vi "Day08-02_모터 속도 변경.vi"() -> ()   [LabVIEW 2021]
uses:
  <vilib>/DAQmx/read.llb/DAQmx Read (Counter DBL 1Chan 1Samp).vi
  <vilib>/DAQmx/write.llb/DAQmx Write (Digital Bool 1Line 1Point).vi
  <vilib>/DAQmx/write.llb/DAQmx Write (Counter Frequency 1Chan 1Samp).vi
  <vilib>/DAQmx/create/channels.llb/DAQmx Create Channel (CO-Pulse Generation-Frequency).vi
  <vilib>/DAQmx/configure/timing.llb/DAQmx Timing (Implicit).vi
  <vilib>/DAQmx/create/channels.llb/DAQmx Create Channel (DO-Digital Output).vi
  <vilib>/DAQmx/create/channels.llb/DAQmx Create Channel (CI-Count Edges).vi
  <vilib>/DAQmx/miscellaneous.llb/DAQmx Fill In Error Info.vi
  <resource>/objmgr/daqmx.rc
panel:
  out "RPM":dbl
  in  "정회전":bool caption="데이터"
  in  "주기 점유율 2":dbl=0.1 min=0.1 max=0.9 step=0.1
  in  "정지 3":bool
  in  "정지 2":bool
  in  "주기 점유율":dbl=0.1 min=0.1 max=0.9 step=0.1
  in  "초기 지연":dbl format="%.6f"
  in  "정지":bool
  in  "주파수":dbl=1.0 format="%.6f"
  in  "주기 점유율":dbl=0.5 format="%.6f"
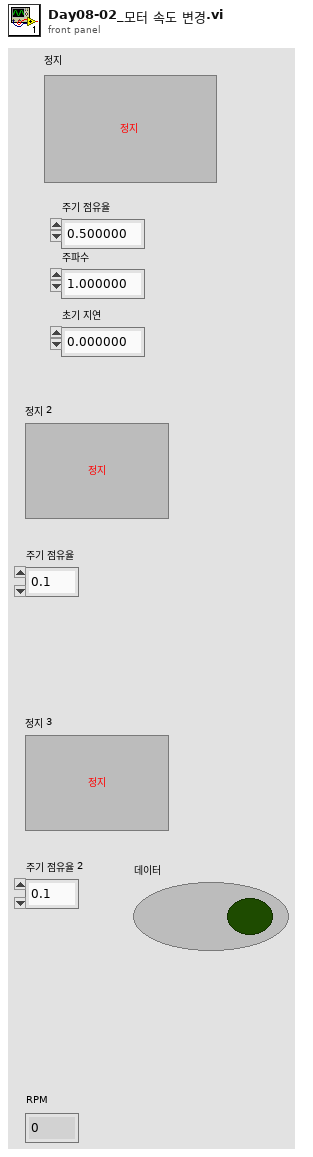
[diagram p1: front panel]
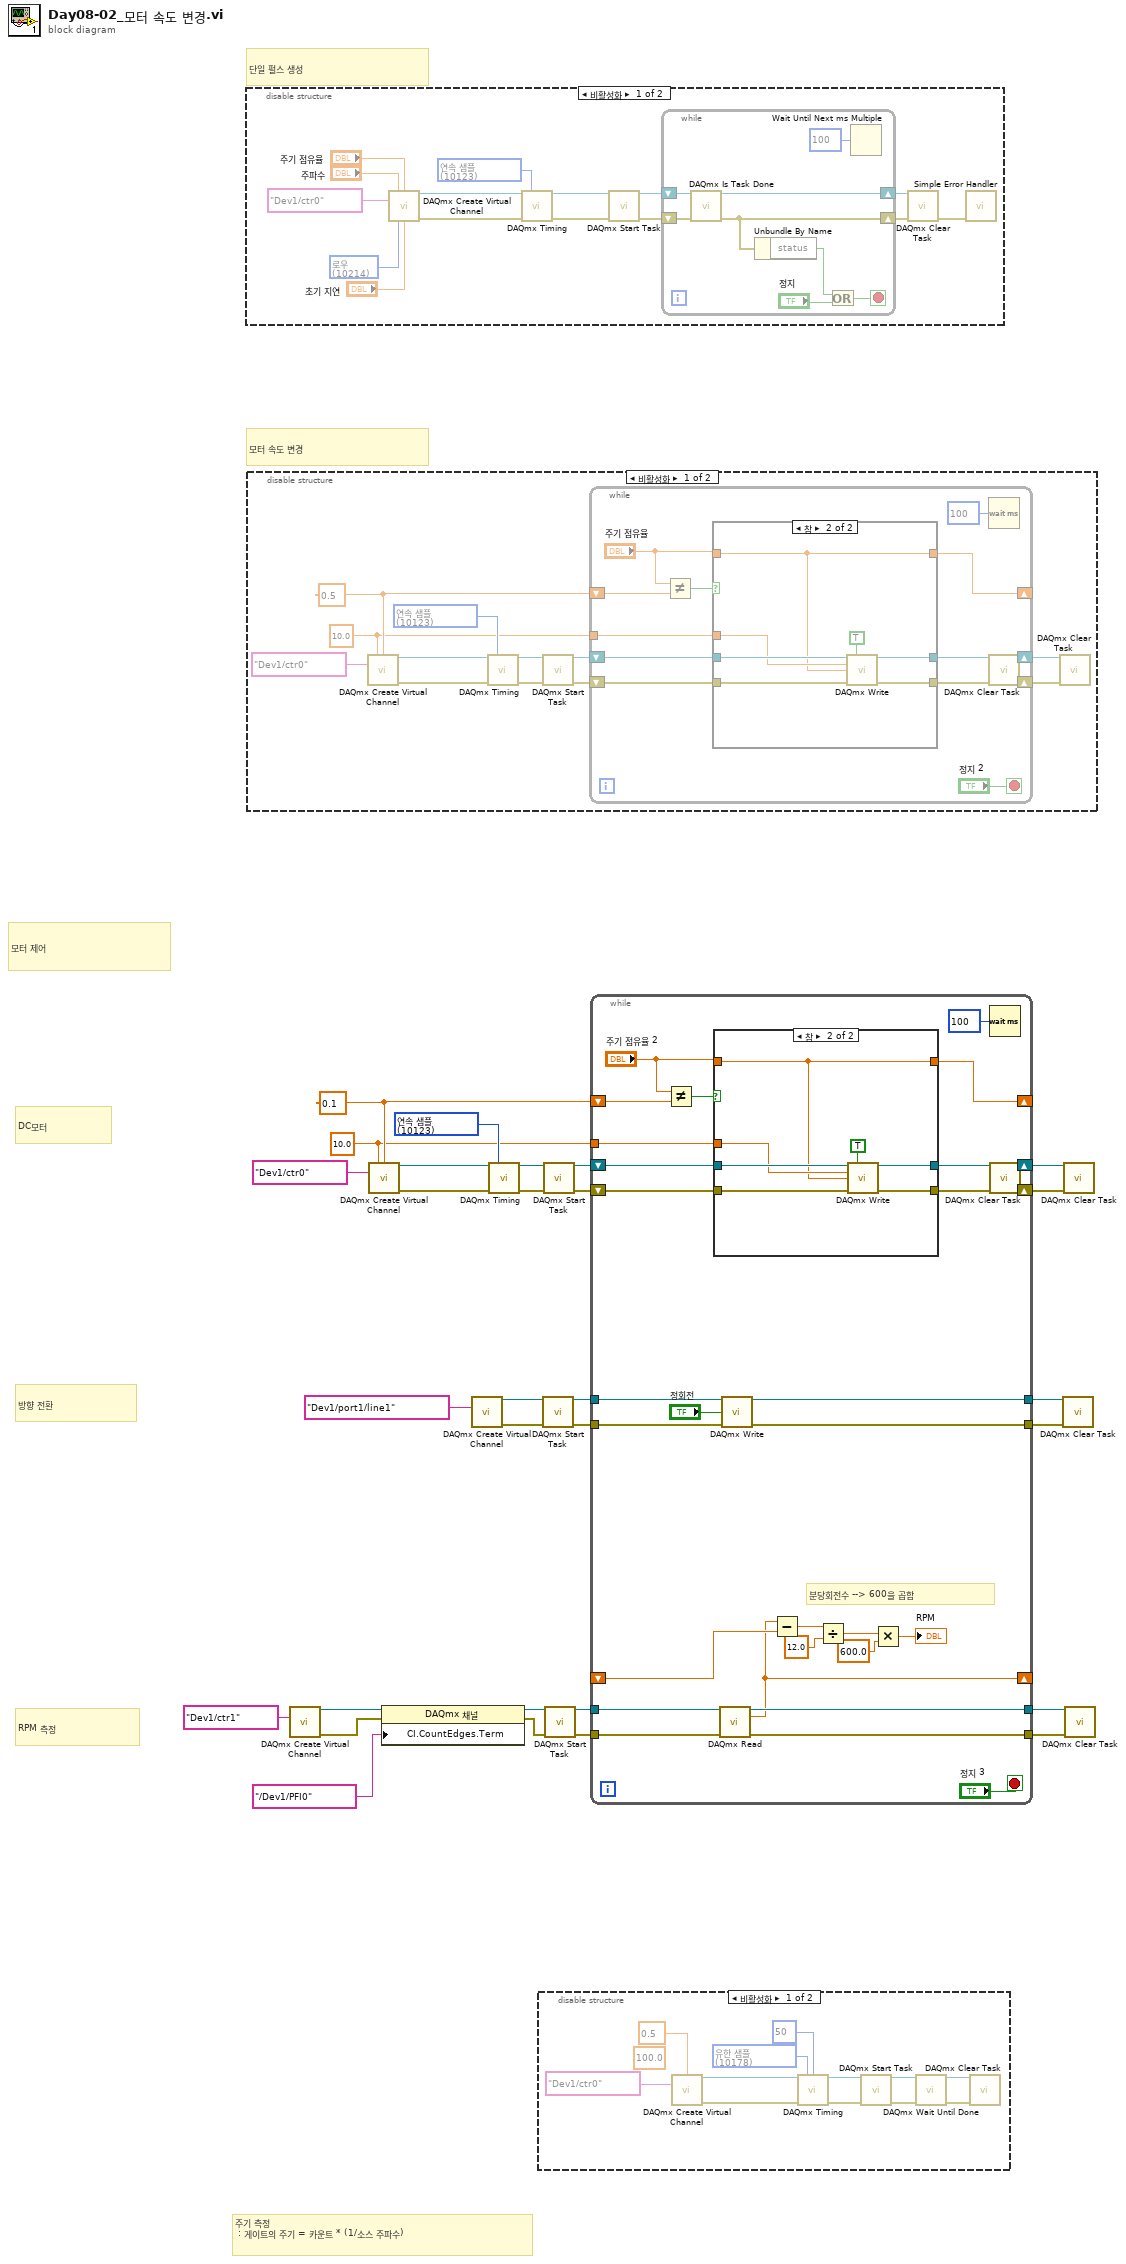
[diagram p0: block diagram]
diagram:
  w18 = 10.0
  w19 = 0.1
  w22 = 10123 items=["유한 샘플"=10178, "연속 샘플"=10123, "하드웨어 타이밍에 의한 단일 포인트"=12522] ("sample mode")
  # "RPM 측정"
  # "방향 전환"
  # "DC모터"
  # "주기 측정\n : 게이트의 주기 = 카운트 * (1/소스 주파수)"
  # "모터 제어"
  # "단일 펄스 생성"
  # "모터 속도 변경"
  n1 = disable-structure shown="비활성화" {
    frame Disabled {
      w34 = 10123 items=["유한 샘플"=10178, "연속 샘플"=10123, "하드웨어 타이밍에 의한 단일 포인트"=12522] ("sample mode")
      w36 = 10214 items=["하이"=10192, "로우"=10214] ("idle state")
      n2 = call-poly <vilib>:"DAQmx Create Virtual Channel.vi"("frequency"="주파수", "duty cycle"="주기 점유율", "counter"=tag "Dev1/ctr0", "idle state"=w36, "initial delay"="초기 지연") -> ("task out"=w44:refnum<k21>, "error out"=w43:errorcluster)  [unwired: 9 in]
      n3 = call-poly <vilib>:"DAQmx Timing.vi"("task/channels in"=w44, "sample mode"=w34, "error in"=w43) -> ("task out"=w42:refnum<k21>, "error out"=w41:errorcluster)  [unwired: 11 in]
      n4 = call <vilib>:"DAQmx Start Task.vi"("task/channels in"=w42, "error in"=w41) -> ("task out"=w40:refnum<k21>, "error out"=w39:errorcluster)  [unwired: 12 in]
      n5 = while {
        shift-right: [w50] -> w38
        shift-left: w40 -> [w52]
        shift-right: [w47] -> w37
        shift-left: w39 -> [w51]
        stop <- w48 stop-if-true
        n6 = call <vilib>:"DAQmx Is Task Done.vi"("task/channels in"=w52, "error in"=w51) -> ("task out"=w50:refnum<k21>, "error out"=w47:errorcluster)  [unwired: 11 in, 1 out]
        n7 = Unbundle By Name(w47) -> ("status"=w46:bool)
        n8 = Or(x=w46, y="정지") -> (x .or. y?=w48:bool)
        n9 = Wait Until Next ms Multiple(millisecond multiple=u32 100 ("ms 배수")) -> ()  [unwired: 1 out]
      }
      n10 = call <vilib>:"DAQmx Clear Task.vi"("task in"=w38, "error in"=w37) -> ("error out"=w33:errorcluster)  [unwired: 13 in]
      n11 = call <vilib>:"Simple Error Handler.vi"("error in (no error)"=w33) -> ()  [unwired: 4 in, 5 out]
    }
    frame Enabled {
    }
  }
  n12 = disable-structure shown="비활성화" {
    frame Disabled {
      w53 = 10.0
      w54 = 0.5
      w57 = 10123 items=["유한 샘플"=10178, "연속 샘플"=10123, "하드웨어 타이밍에 의한 단일 포인트"=12522] ("sample mode")
      n13 = call-poly <vilib>:"DAQmx Create Virtual Channel.vi"("frequency"=w53, "duty cycle"=w54, "counter"=tag "Dev1/ctr0") -> ("task out"=w64:refnum<k21>, "error out"=w63:errorcluster)  [unwired: 11 in]
      n14 = call-poly <vilib>:"DAQmx Timing.vi"("task/channels in"=w64, "sample mode"=w57, "error in"=w63) -> ("task out"=w62:refnum<k21>, "error out"=w61:errorcluster)  [unwired: 11 in]
      n15 = call <vilib>:"DAQmx Start Task.vi"("task/channels in"=w62, "error in"=w61) -> ("task out"=w60:refnum<k21>, "error out"=w59:errorcluster)  [unwired: 12 in]
      n16 = while {
        shift-right: [w73] -> w56
        shift-left: w60 -> [w75]
        shift-right: [w72] -> w55
        shift-left: w59 -> [w74]
        shift-right: [w65] -> _
        shift-left: w54 -> [w68]
        tunnel: w53 -> [w70]
        stop <- "정지 2" stop-if-true
        n17 = Not Equal?(x="주기 점유율", y=w68) -> (x != y?=w69:bool)
        n18 = case shown="참" w69 {
          tunnel: w75 -> [w77 w85]
          tunnel: w74 -> [w76 w84]
          tunnel: [w77 w83] -> w73
          tunnel: [w76 w82] -> w72
          tunnel: w70 -> [_ w80]
          tunnel: "주기 점유율" -> [w78 w79]
          tunnel: [w78 w79] -> w65
          frame False {
          }
          frame True {
            n19 = call-poly <vilib>:"DAQmx Write.vi"("task/channels in"=w85, "auto start"=TRUE, "frequency"=w80, "duty cycle"=w79, "error in"=w84) -> ("task out"=w83:refnum<k21>, "error out"=w82:errorcluster)  [unwired: 8 in, 1 out]
          }
        }
        n20 = Wait (ms)(milliseconds to wait=u32 100 ("대기 시간 (ms)")) -> ()  [unwired: 1 out]
      }
      n21 = call <vilib>:"DAQmx Clear Task.vi"("task in"=w56, "error in"=w55) -> ()  [unwired: 13 in, 1 out]
      n22 = call <vilib>:"DAQmx Clear Task.vi"("task in"=w56, "error in"=w55) -> ()  [unwired: 13 in, 1 out]
    }
    frame Enabled {
    }
  }
  n23 = call-poly <vilib>:"DAQmx Create Virtual Channel.vi"("counter"=tag "Dev1/ctr1") -> ("task out"=w10:refnum<k21>, "error out"=w3:errorcluster)  [unwired: 13 in]
  n24 = call-poly <vilib>:"DAQmx Create Virtual Channel.vi"("frequency"=w18, "duty cycle"=w19, "counter"=tag "Dev1/ctr0") -> ("task out"=w29:refnum<k21>, "error out"=w28:errorcluster)  [unwired: 11 in]
  n25 = property class="DAQmx 채널"(reference=w10, error in=w3, "CI.CountEdges.Term"=tag "/Dev1/PFI0" ("카운터 입력:에지 카운트:입력:터미널")) -> (reference out=w5:refnum<k21>, error out=w2:errorcluster)
  n26 = call-poly <vilib>:"DAQmx Create Virtual Channel.vi"("lines"=tag "Dev1/port1/line1") -> ("task out"=w17:refnum<k21>, "error out"=w16:errorcluster)  [unwired: 13 in]
  n27 = call-poly <vilib>:"DAQmx Timing.vi"("task/channels in"=w29, "sample mode"=w22, "error in"=w28) -> ("task out"=w27:refnum<k21>, "error out"=w26:errorcluster)  [unwired: 11 in]
  n28 = disable-structure shown="비활성화" {
    frame Disabled {
      w87 = 10178 items=["유한 샘플"=10178, "연속 샘플"=10123, "하드웨어 타이밍에 의한 단일 포인트"=12522] ("sample mode")
      (unwired) 100.0 ("maximum value")
      n29 = call-poly <vilib>:"DAQmx Create Virtual Channel.vi"("duty cycle"=0.5 ("minimum value"), "counter"=tag "Dev1/ctr0") -> ("task out"=w89:refnum<k21>, "error out"=w88:errorcluster)  [unwired: 12 in]
      n30 = call-poly <vilib>:"DAQmx Timing.vi"("task/channels in"=w89, "sample mode"=w87, "samples per channel"=50, "error in"=w88) -> ("task out"=w97:refnum<k21>, "error out"=w96:errorcluster)  [unwired: 10 in]
      n31 = call <vilib>:"DAQmx Start Task.vi"("task/channels in"=w97, "error in"=w96) -> ("task out"=w95:refnum<k21>, "error out"=w94:errorcluster)  [unwired: 12 in]
      n32 = call <vilib>:"DAQmx Wait Until Done.vi"("task/channels in"=w95, "error in"=w94) -> ("task out"=w93:refnum<k21>, "error out"=w92:errorcluster)  [unwired: 12 in]
      n33 = call <vilib>:"DAQmx Clear Task.vi"("task in"=w93, "error in"=w92) -> ()  [unwired: 13 in, 1 out]
    }
    frame Enabled {
    }
  }
  n34 = call <vilib>:"DAQmx Start Task.vi"("task/channels in"=w17, "error in"=w16) -> ("task out"=w15:refnum<k21>, "error out"=w14:errorcluster)  [unwired: 12 in]
  n35 = call <vilib>:"DAQmx Start Task.vi"("task/channels in"=w27, "error in"=w26) -> ("task out"=w25:refnum<k21>, "error out"=w24:errorcluster)  [unwired: 12 in]
  n36 = call <vilib>:"DAQmx Start Task.vi"("task/channels in"=w5, "error in"=w2) -> ("task out"=w9:refnum<k21>, "error out"=w8:errorcluster)  [unwired: 12 in]
  n37 = while {
    shift-right: [w122] -> w21
    shift-left: w25 -> [w124]
    shift-right: [w121] -> w20
    shift-left: w24 -> [w123]
    shift-right: [w114] -> _
    shift-left: w19 -> [w117]
    tunnel: w18 -> [w119]
    tunnel: w15 -> [w113]
    tunnel: w14 -> [w112]
    tunnel: [w111] -> w13
    tunnel: [w110] -> w12
    tunnel: w9 -> [w108]
    tunnel: w8 -> [w107]
    tunnel: [w106] -> w7
    tunnel: [w105] -> w6
    shift-right: [w98] -> _
    shift-left: _ -> [w99]
    stop <- "정지 3" stop-if-true
    # "분당회전수 --> 600을 곱함"
    n38 = Not Equal?(x="주기 점유율 2", y=w117) -> (x != y?=w118:bool)
    n39 = case shown="참" w118 {
      tunnel: w124 -> [w126 w134]
      tunnel: w123 -> [w125 w133]
      tunnel: [w126 w132] -> w122
      tunnel: [w125 w131] -> w121
      tunnel: w119 -> [_ w129]
      tunnel: "주기 점유율 2" -> [w127 w128]
      tunnel: [w127 w128] -> w114
      frame False {
      }
      frame True {
        n40 = call-poly <vilib>:"DAQmx Write.vi"("task/channels in"=w134, "auto start"=TRUE, "frequency"=w129, "duty cycle"=w128, "error in"=w133) -> ("task out"=w132:refnum<k21>, "error out"=w131:errorcluster)  [unwired: 8 in, 1 out]
      }
    }
    n41 = call-poly <vilib>:"DAQmx Read.vi"("task/channels in"=w108, "error in"=w107) -> ("task out"=w106:refnum<k21>, "data"=w98:dbl, "error out"=w105:errorcluster)  [unwired: 11 in]
    n42 = call-poly <vilib>:"DAQmx Write.vi"("task/channels in"=w113, "data"="정회전", "error in"=w112) -> ("task out"=w111:refnum<k21>, "error out"=w110:errorcluster)  [unwired: 10 in, 1 out]
    n43 = Subtract(x=w98, y=w99) -> (x-y=w104:dbl)
    n44 = Divide(x=w104, y=12.0) -> (x/y=w102:dbl)
    n45 = Multiply(x=w102, y=600.0) -> (x*y=→"RPM":dbl)
    n46 = Wait (ms)(milliseconds to wait=u32 100 ("대기 시간 (ms)")) -> ()  [unwired: 1 out]
  }
  n47 = call <vilib>:"DAQmx Clear Task.vi"("task in"=w21, "error in"=w20) -> ()  [unwired: 13 in, 1 out]
  n48 = call <vilib>:"DAQmx Clear Task.vi"("task in"=w13, "error in"=w12) -> ()  [unwired: 13 in, 1 out]
  n49 = call <vilib>:"DAQmx Clear Task.vi"("task in"=w21, "error in"=w20) -> ()  [unwired: 13 in, 1 out]
  n50 = call <vilib>:"DAQmx Clear Task.vi"("task in"=w7, "error in"=w6) -> ()  [unwired: 13 in, 1 out]
